vi "Position First String.vi"(6 "Units":refnum<vi>, 8 "error in (no error)":errorcluster, 10 "Button Ref":refnum<vi>, 11 "String Ref":refnum<vi>) -> (0 "Error Out":errorcluster)   [LabVIEW 2014]
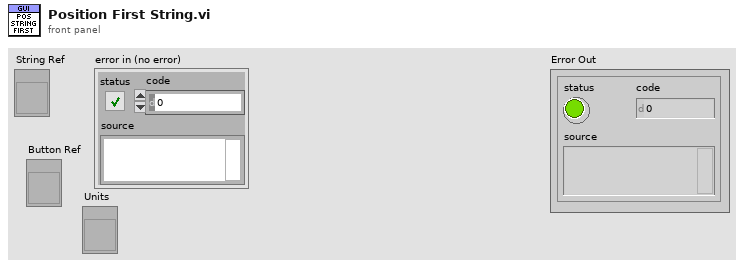
[diagram p1: front panel]
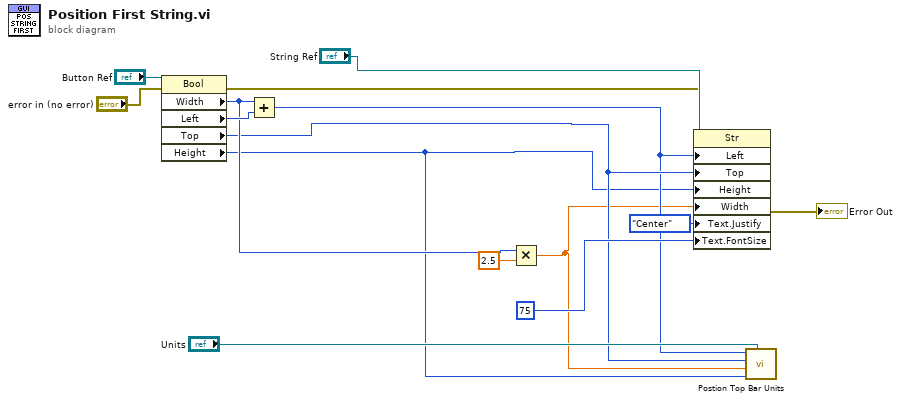
[diagram p0: block diagram]
diagram:
  n1 = property class="Bool"(reference="Button Ref", error in="error in (no error)") -> (error out=w8:errorcluster, "Width"=w11:u32, "Left"=w13:i32, "Top"=w4:i32, "Height"=w2:u32)  [unwired: 1 out]
  n2 = Add(x=w11, y=w13) -> (x+y=w3:u32)
  n3 = Multiply(x=w11, y=2.5) -> (x*y=w1:dbl)
  n4 = property class="Str"(reference="String Ref", error in=w8, "Left"=w3, "Top"=w4, "Height"=w2, "Width"=w1, "Text.Justify"=enum16{"Left", "Center", "Right"}."Center" ("Text.Justification"), "Text.FontSize"=u32 75 ("Text.Font:Size")) -> (error out=→"Error Out":errorcluster)  [unwired: 1 out]
  n5 = call "Postion Top Bar Units.vi"("Units"="Units", "Button Size:Height"=w2, "Button Witdh"=w1, "Top (numeric indicator)"=w4, "Left (numeric indicator)"=w3) -> ()  [unwired: 6 in, 1 out]
